vi "kuvaitech.vi"() -> ()   [LabVIEW 2021]
panel:
  in  "Numeric":dbl
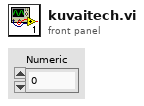
[diagram p1: front panel]
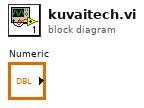
[diagram p0: block diagram]
diagram:
